vi "Setup UI.vi"(8 "error in (no error)":errorcluster, 10 "Set UI to input? (F)":bool, 11 "Pulse Gen Basic Scan in":refnum<class "Pulse Gen Basic Scan.lvclass">) -> (0 "error out":errorcluster, 3 "Pulse Gen Basic Scan out":refnum<class "Pulse Gen Basic Scan.lvclass">)   [LabVIEW 2009, in "Pulse Gen Basic Scan.lvclass"]
doc: "Scanner::Setup is a constructor that has no parameters and faces the user. The Factory calls this VI to let the user configure this Scanner. It is dynamically dispatched in order to let the user choose the type as well as the options of the scanner."
uses:
  Pulse Gen Basic Scan.lvclass
  Pulse Gen Basic Scan.lvclass/Pulse Gen Basic Scan.ctl
panel:
  in  "Overall Frequency":dbl[unit]
  in  "period/frequency":bool
  in  "Send conds for first point to PG":bool
  in  "Ch2Width ind variable?":bool
  in  "Ch2Delay ind variable?":bool
  in  "Ch1Width ind variable?":bool
  in  "Ch1Delay ind variable?":bool
  in  "Ch2Width":dbl[unit]
  in  "Ch2Delay":dbl[unit]
  in  "Ch1Width":dbl[unit]
  in  "Ch1Delay":dbl[unit]
  in  "Overall Period":dbl[unit]
  # "Pulse Gen Basic Scan"
  # "Pulse Gen Basic Scan: This forces the PG to CONTINUOUS PULSES mode, and allowes the user to vary only the basic settings that could be changed from the front panel. \nNote: independent variable must be in ns."
  # "ind. variable?"
  # "Desired overall period/frequency"
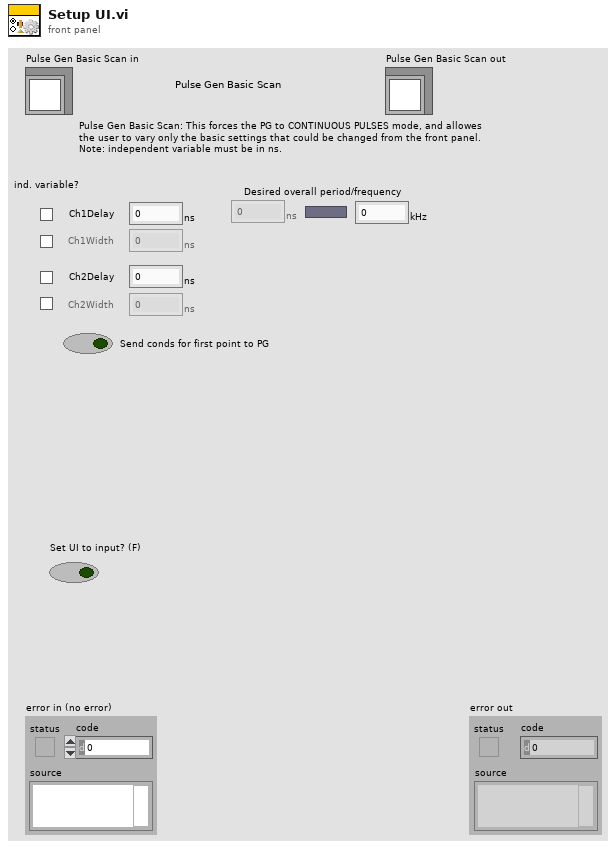
[diagram p1: front panel]
types:
  T1 = enum8{"Enabled", "Disabled", "Disabled and Grayed Out"}
  T2 = typedef "Scanner.lvclass/Range.ctl" = cluster{"xi":dbl, "xf":dbl, "dx":dbl, "Return to...?":bool, "Return to":dbl}
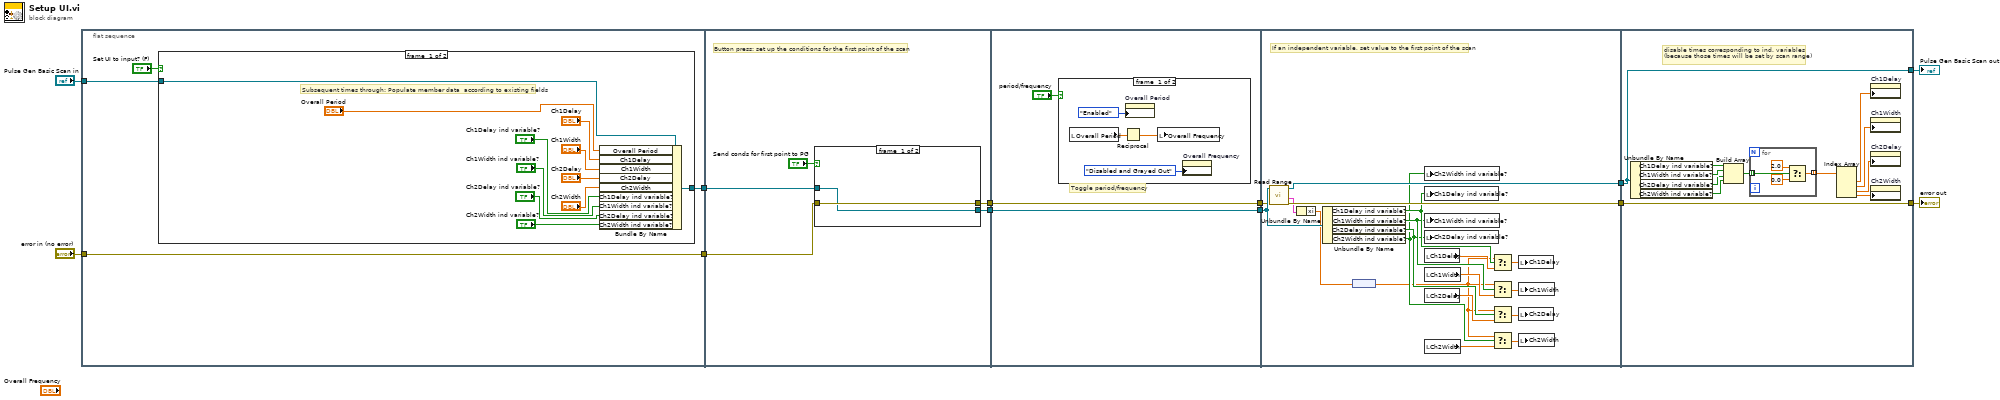
[diagram p0: block diagram]
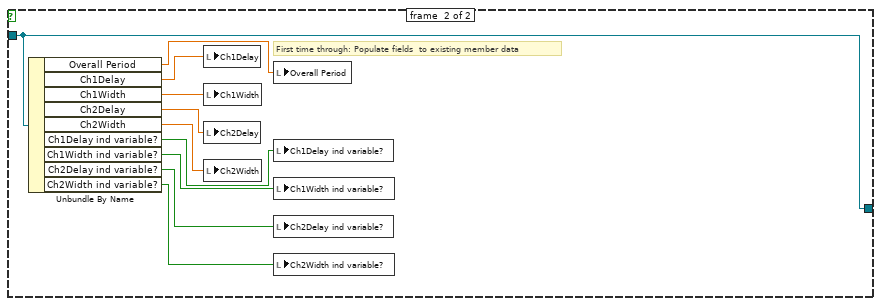
[diagram p2: hidden frame]
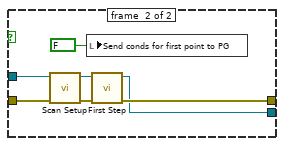
[diagram p3: hidden frame]
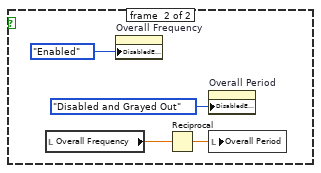
[diagram p4: hidden frame]
diagram:
  n1 = flat-sequence {
    tunnel: "error in (no error)" -> [w16]
    tunnel: "Pulse Gen Basic Scan in" -> [w14]
    tunnel: [w16] -> w9
    tunnel: [w13] -> w8
    tunnel: w9 -> [w41]
    tunnel: w8 -> [w39]
    tunnel: [w40] -> w6
    tunnel: [w38] -> w5
    tunnel: w6 -> [w54]
    tunnel: w5 -> [w53]
    tunnel: [w54] -> w4
    tunnel: [w53] -> w3
    tunnel: w4 -> [w79]
    tunnel: w3 -> [w81]
    tunnel: [w78] -> w2
    tunnel: [w80] -> w1
    tunnel: [w87] -> w7
    tunnel: [w93] -> w12
    tunnel: w2 -> [w93]
    tunnel: w1 -> [w87]
    frame #0 {
      n2 = case shown="False" "Set UI to input? (F)" {
        tunnel: w14 -> [w27 w28]
        tunnel: [w17 w28] -> w13
        frame #0 {
          # "Subsequent times through: Populate member data  according to existing fields"
          n3 = Bundle By Name(cluster=w27, "Overall Period"="Overall Period", "Ch1Delay"="Ch1Delay", "Ch1Width"="Ch1Width", "Ch2Delay"="Ch2Delay", "Ch2Width"="Ch2Width", "Ch1Delay ind variable?"="Ch1Delay ind variable?", "Ch1Width ind variable?"="Ch1Width ind variable?", "Ch2Delay ind variable?"="Ch2Delay ind variable?", "Ch2Width ind variable?"="Ch2Width ind variable?") -> (w17:refnum<class "Pulse Gen Basic Scan.lvclass">)
        }
        frame #1 {
          # "First time through: Populate fields  to existing member data"
          n4 = Unbundle By Name(w28) -> ("Overall Period"=w37:dbl[unit], "Ch1Delay"=w35:dbl[unit], "Ch1Width"=w36:dbl[unit], "Ch2Delay"=w34:dbl[unit], "Ch2Width"=w33:dbl[unit], "Ch1Delay ind variable?"=w32:bool, "Ch1Width ind variable?"=w31:bool, "Ch2Delay ind variable?"=w30:bool, "Ch2Width ind variable?"=w29:bool)
          n5 = local write "Ch1Delay"(w35) -> ()
          n6 = local write "Ch1Width"(w36) -> ()
          n7 = local write "Ch2Delay"(w34) -> ()
          n8 = local write "Ch2Width"(w33) -> ()
          n9 = local write "Overall Period"(w37) -> ()
          n10 = local write "Ch1Delay ind variable?"(w32) -> ()
          n11 = local write "Ch1Width ind variable?"(w31) -> ()
          n12 = local write "Ch2Delay ind variable?"(w30) -> ()
          n13 = local write "Ch2Width ind variable?"(w29) -> ()
        }
      }
    }
    frame #1 {
      # "Button press: set up the conditions for the first point of the scan"
      n14 = case shown="True" "Send conds for first point to PG" {
        tunnel: w41 -> [w44 w50]
        tunnel: [w44 w48] -> w40
        tunnel: w39 -> [w43 w47]
        tunnel: [w43 w45] -> w38
        frame #0 {
        }
        frame #1 {
          n15 = call-dynamic "Scan Setup.vi"("error in (no error)"=w50, "Pulse Gen Basic Scan in"=w47) -> ("error out"=w49:errorcluster, "Pulse Gen Basic Scan out"=w46:refnum<class "Pulse Gen Basic Scan.lvclass">)  [unwired: 8 in]
          n16 = local write "Send conds for first point to PG"(FALSE ("Send conds for first point to PG")) -> ()
          n17 = call-dynamic "First Step.vi"("error in (no error)"=w49, "Pulse Gen Basic Scan.lvclass in"=w46) -> ("error out"=w48:errorcluster, "Pulse Gen Basic Scan.lvclass out"=w45:refnum<class "Pulse Gen Basic Scan.lvclass">)  [unwired: 7 in, 1 out]
        }
      }
    }
    frame #2 {
      # "Toggle period/frequency"
      n18 = case shown="False" "period/frequency" {
        frame #0 {
          n19 = local read "Overall Period"() -> (w58:dbl[unit])
          n20 = Reciprocal(x=w58) -> (1/x=w57:dbl[unit])
          n21 = property on="Overall Period" class="DigNum (strict)"("DisabledEnum"=T1."Enabled" ("Disabled")) -> ()  [unwired: 2 in, 2 out]
          n22 = local write "Overall Frequency"(w57) -> ()
          n23 = property on="Overall Frequency" class="DigNum (strict)"("DisabledEnum"=T1."Disabled and Grayed Out" ("Disabled")) -> ()  [unwired: 2 in, 2 out]
        }
        frame #1 {
          n24 = local read "Overall Frequency"() -> (w60:dbl[unit])
          n25 = property on="Overall Frequency" class="DigNum (strict)"("DisabledEnum"=T1."Enabled" ("Disabled")) -> ()  [unwired: 2 in, 2 out]
          n26 = Reciprocal(x=w60) -> (1/x=w59:dbl[unit])
          n27 = property on="Overall Period" class="DigNum (strict)"("DisabledEnum"=T1."Disabled and Grayed Out" ("Disabled")) -> ()  [unwired: 2 in, 2 out]
          n28 = local write "Overall Period"(w59) -> ()
        }
      }
    }
    frame #3 {
      # "If an independent variable, set value to the first point of the scan"
      n29 = call-dynamic "Read Range.vi"("error in (no error)"=w79, "Scanner.lvclass in"=w81) -> ("error out"=w78:errorcluster, "Range"=w77:T2, "Scanner.lvclass out"=w80:refnum<class "Pulse Gen Basic Scan.lvclass">)  [unwired: 7 out]
      n30 = Unbundle By Name(w77) -> ("xi"=w64:dbl)
      n31 = Unbundle By Name(w81) -> ("Ch1Delay ind variable?"=w68:bool, "Ch1Width ind variable?"=w67:bool, "Ch2Delay ind variable?"=w66:bool, "Ch2Width ind variable?"=w65:bool)
      n32 = node(w64) -> (w63:dbl[unit])
      n33 = local write "Ch2Width ind variable?"(w65) -> ()
      n34 = local write "Ch1Delay ind variable?"(w68) -> ()
      n35 = local write "Ch1Width ind variable?"(w67) -> ()
      n36 = local write "Ch2Delay ind variable?"(w66) -> ()
      n37 = local read "Ch1Delay"() -> (w69:dbl[unit])
      n38 = local read "Ch1Width"() -> (w70:dbl[unit])
      n39 = local read "Ch2Delay"() -> (w71:dbl[unit])
      n40 = local read "Ch2Width"() -> (w72:dbl[unit])
      n41 = Select(t=w63, s=w68, f=w69) -> (s? t:f=w76:dbl[unit])
      n42 = Select(t=w63, s=w67, f=w70) -> (s? t:f=w75:dbl[unit])
      n43 = Select(t=w63, s=w66, f=w71) -> (s? t:f=w74:dbl[unit])
      n44 = Select(t=w63, s=w65, f=w72) -> (s? t:f=w73:dbl[unit])
      n45 = local write "Ch1Delay"(w76) -> ()
      n46 = local write "Ch1Width"(w75) -> ()
      n47 = local write "Ch2Delay"(w74) -> ()
      n48 = local write "Ch2Width"(w73) -> ()
    }
    frame #4 {
      # "disable times corresponding to ind. variables \n(because those times will be set by scan range)"
      n49 = Unbundle By Name(w87) -> ("Ch1Delay ind variable?"=w86:bool, "Ch1Width ind variable?"=w85:bool, "Ch2Delay ind variable?"=w84:bool, "Ch2Width ind variable?"=w83:bool)
      n50 = Build Array(w86, w85, w84, w83) -> (w82:bool[])
      n51 = for {
        tunnel: [w95] -> w92 mode=indexing
        tunnel: w82 -> [w94] mode=indexing
        n52 = Select(t=2.0, s=w94, f=0.0) -> (s? t:f=w95:dbl)
      }
      n53 = Index Array(array=w92) -> (element #1=w91:dbl, element #2=w90:dbl, element #3=w89:dbl, element #4=w88:dbl)  [unwired: 4 in]
      n54 = property on="Ch1Delay" class="DigNum (strict)"("DisabledEnum"=w91) -> ()  [unwired: 2 in, 2 out]
      n55 = property on="Ch1Width" class="DigNum (strict)"("DisabledEnum"=w90) -> ()  [unwired: 2 in, 2 out]
      n56 = property on="Ch2Delay" class="DigNum (strict)"("DisabledEnum"=w89) -> ()  [unwired: 2 in, 2 out]
      n57 = property on="Ch2Width" class="DigNum (strict)"("DisabledEnum"=w88) -> ()  [unwired: 2 in, 2 out]
    }
  }
  "error out" <- w12
  "Pulse Gen Basic Scan out" <- w7
